vi "Pre-Process.vi"(11 "Ship in":refnum<class "Ship.lvclass">) -> (3 "Ship out":refnum<class "Ship.lvclass">)   [LabVIEW 2021, in "Ship.lvclass"]
uses:
  Ship.lvclass
  Element/Element.lvclass
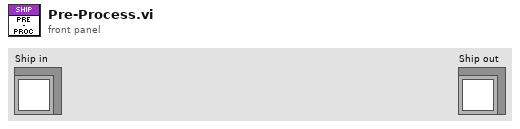
[diagram p1: front panel]
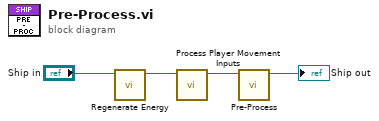
[diagram p0: block diagram]
diagram:
  n1 = call "Regenerate Energy.vi"("Ship in"="Ship in") -> ("Ship out"=w1:refnum<class "Ship.lvclass">)  [unwired: 10 in]
  n2 = call "Process Player Movement Inputs.vi"("Ship in"=w1) -> ("Ship out"=w4:refnum<class "Ship.lvclass">)  [unwired: 10 in]
  n3 = call-parent "Pre-Process.vi"("Element in"=w4) -> ("Element out"=→"Ship out":refnum<class "Ship.lvclass">)  [unwired: 10 in]
